vi "Line Settings FGV.vi"(8 "error in (no error)":errorcluster, 9 "Get/Set":enum16{"Set", "Get"}(ring), 10 "Line":T1={"Topic Name"="MyTopic", "Domain Id"=0, "Advanced Configuration"={"typeName"="", "key Name"=enum."<none>", "domainParticipantQoSProfile"="", "dataWriterQoSProfile"="", "forceArrayMapping?"=FALSE, "forceUnboundedString?"=FALSE, "forceExclusiveReader?"=FALSE, "forceRead? (only ExclusiveReader)"=FALSE, "ContentFilteredTopic Info"={"Filter Type"="DDS_SQLFILTER_NAME", "ContentFilteredTopic Name"="", "Filter Expression"=""}}}, 11 "Item Ref in":T5 format="%.0x") -> (0 "error out":errorcluster, 2 "Line":T1={"Topic Name"="MyTopic", "Domain Id"=0, "Advanced Configuration"={"typeName"="", "key Name"=enum."<none>", "domainParticipantQoSProfile"="", "dataWriterQoSProfile"="", "forceArrayMapping?"=FALSE, "forceUnboundedString?"=FALSE, "forceExclusiveReader?"=FALSE, "forceRead? (only ExclusiveReader)"=FALSE, "ContentFilteredTopic Info"={"Filter Type"="DDS_SQLFILTER_NAME", "ContentFilteredTopic Name"="", "Filter Expression"=""}}}, 3 "Item Ref out":T5=18446744073709551615 format="%.0x")   [LabVIEW 2016, in "DDS Custom Device System Explorer.lvlib"]
uses:
  DDS Custom Device System Explorer.lvlib
  <vilib>/NI Veristand/Custom Device API/Custom Device Item Ref.ctl
  Shared/WriterReaderConfiguration.ctl
  Shared/Advanced DDS Configuration.ctl
  Shared/key Enum.ctl
  <vilib>/RTI DDS Toolkit/Types/RTI DDS ContentFilteredTopic Info.ctl
  Shared/Constants.vi
  <vilib>/NI Veristand/Custom Device API/Set Item Property (U32).vi
  <vilib>/NI Veristand/Custom Device API/Set Item Property (String).vi
  <vilib>/NI Veristand/Custom Device API/Set Item Property (Boolean).vi
  <vilib>/NI Veristand/Custom Device API/Get Item Property (U32).vi
  <vilib>/NI Veristand/Custom Device API/Get Item Property (String).vi
  <vilib>/NI Veristand/Custom Device API/Get Item Property (Boolean).vi
  <vilib>/NI VeriStand/Custom Device API/Custom Device API.lvlib
  Shared/DDS Custom Device Shared.lvlib
  <vilib>/RTI DDS Toolkit/Library/LVDDS_library.lvlib
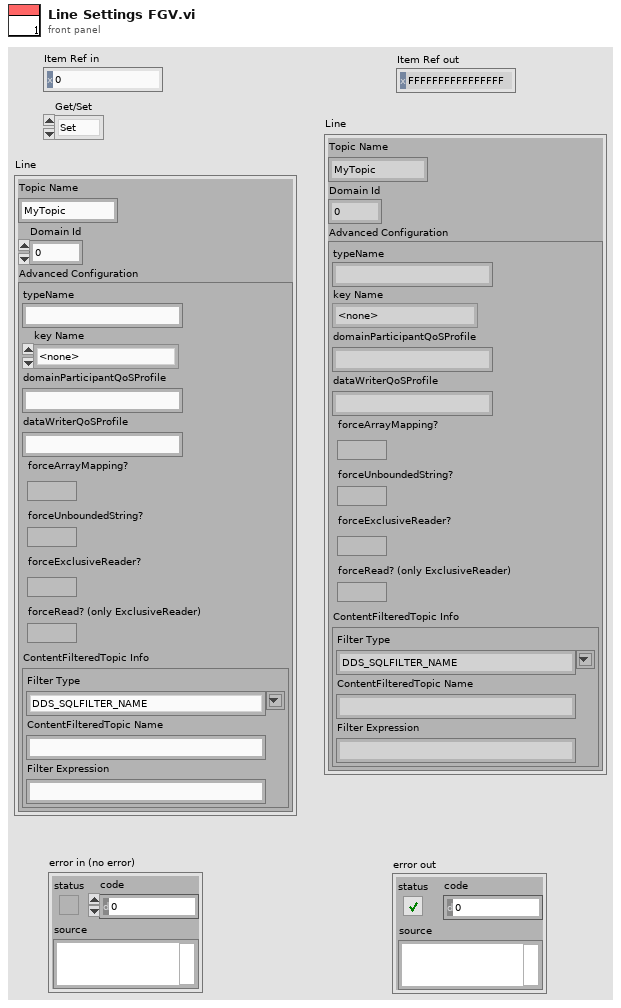
[diagram p1: front panel]
types:
  T1 = typedef "DDS Custom Device Shared.lvlib/WriterReaderConfiguration.ctl" = cluster{"Topic Name":string, "Domain Id":u32, "Advanced Configuration":T2}
  T2 = typedef "DDS Custom Device Shared.lvlib/Advanced DDS Configuration.ctl" = cluster{"typeName":string, "key Name":T3, "domainParticipantQoSProfile":string, "dataWriterQoSProfile":string, "forceArrayMapping?":bool, "forceUnboundedString?":bool, "forceExclusiveReader?":bool, "forceRead? (only ExclusiveReader)":bool, "ContentFilteredTopic Info":T4}
  T3 = typedef "DDS Custom Device Shared.lvlib/key Enum.ctl" = enum16{"<none>", "I32_Num", "I64_Num", "U16_Num", "innercluster.Sgl_Num", "innercluster.Boolean"}
  T4 = typedef "LVDDS_library.lvlib/RTI DDS ContentFilteredTopic Info.ctl" = cluster{"Filter Type":string, "ContentFilteredTopic Name":string, "Filter Expression":string}
  T5 = typedef "Custom Device API.lvlib/Custom Device Item Ref.ctl" = u64
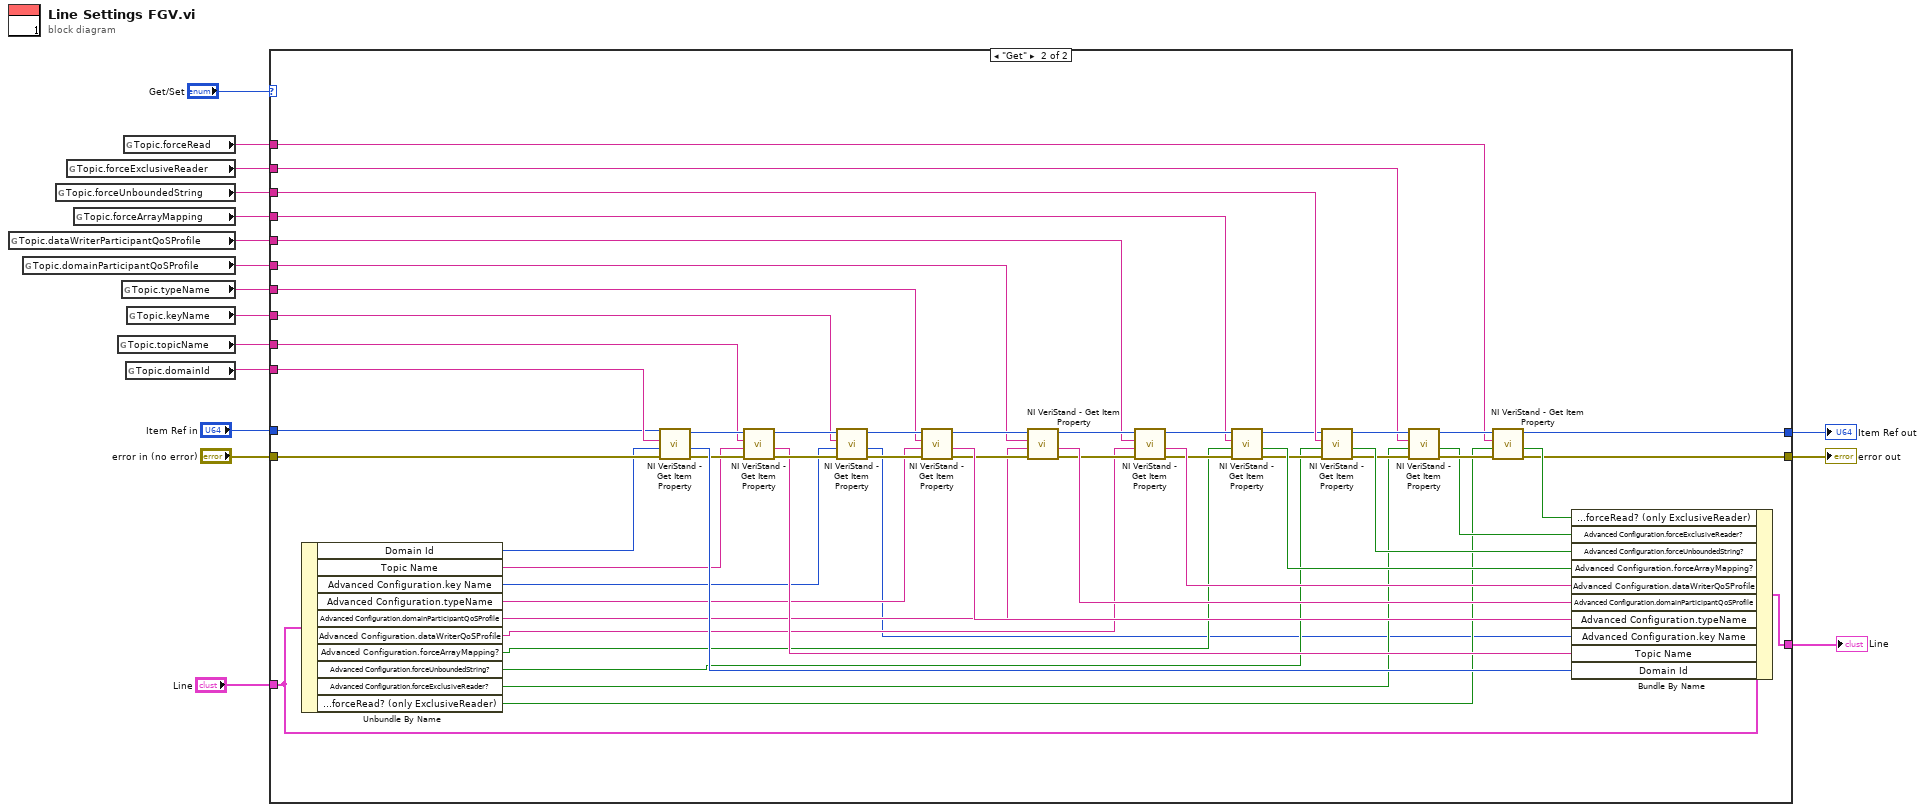
[diagram p0: block diagram]
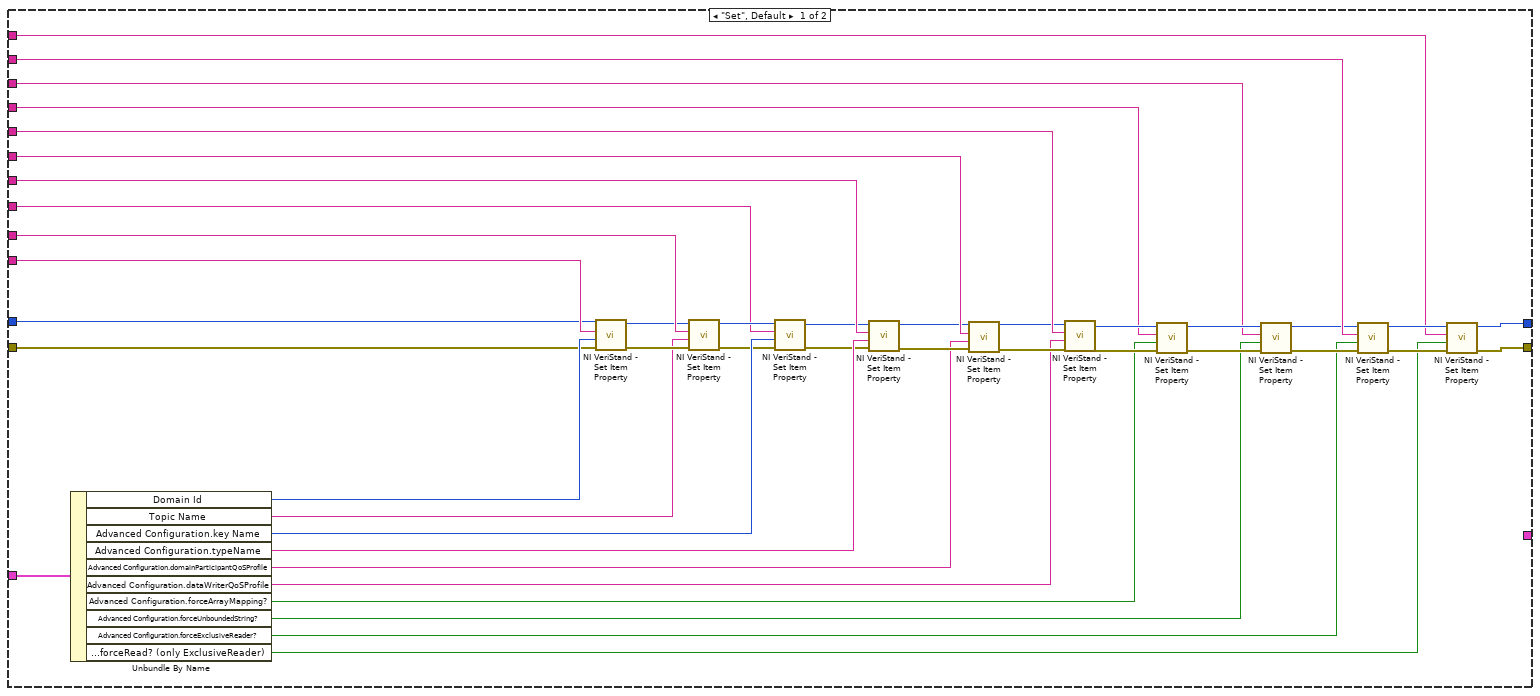
[diagram p2: hidden frame]
diagram:
  n1 = global read "Constants.vi" "Topic.dataWriterParticipantQoSProfile"() -> (w10:string)
  n2 = global read "Constants.vi" "Topic.domainParticipantQoSProfile"() -> (w11:string)
  n3 = global read "Constants.vi" "Topic.forceUnboundedString"() -> (w8:string)
  n4 = global read "Constants.vi" "Topic.forceExclusiveReader"() -> (w4:string)
  n5 = global read "Constants.vi" "Topic.forceArrayMapping"() -> (w9:string)
  n6 = global read "Constants.vi" "Topic.topicName"() -> (w14:string)
  n7 = global read "Constants.vi" "Topic.typeName"() -> (w13:string)
  n8 = global read "Constants.vi" "Topic.forceRead"() -> (w3:string)
  n9 = global read "Constants.vi" "Topic.domainId"() -> (w15:string)
  n10 = global read "Constants.vi" "Topic.keyName"() -> (w5:string)
  n11 = case shown="\"Get\"" "Get/Set" {
    tunnel: "error in (no error)" -> [w18 w73]
    tunnel: w15 -> [w60 w114]
    tunnel: w14 -> [w58 w110]
    tunnel: w13 -> [w57 w103]
    tunnel: "Item Ref in" -> [w19 w74]
    tunnel: w11 -> [w55 w99]
    tunnel: "Line" -> [w52 w72]
    tunnel: w10 -> [w47 w95]
    tunnel: w9 -> [w39 w91]
    tunnel: w8 -> [w38 w88]
    tunnel: [w25 w76] -> w6
    tunnel: [w26 w75] -> w7
    tunnel: w5 -> [w30 w106]
    tunnel: [_ w86] -> w1
    tunnel: w4 -> [w29 w80]
    tunnel: w3 -> [w21 w78]
    frame "Set", Default {
      n12 = Unbundle By Name(w52) -> ("Domain Id"=w51:u32, "Topic Name"=w50:string, "Advanced Configuration.key Name"=w35:T3, "Advanced Configuration.typeName"=w49:string, "Advanced Configuration.domainParticipantQoSProfile"=w48:string, "Advanced Configuration.dataWriterQoSProfile"=w44:string, "Advanced Configuration.forceArrayMapping?"=w37:bool, "Advanced Configuration.forceUnboundedString?"=w36:bool, "Advanced Configuration.forceExclusiveReader?"=w22:bool, "Advanced Configuration.forceRead? (only ExclusiveReader)"=w20:bool)
      n13 = call-poly <vilib>:"NI VeriStand - Set Item Property.vi"("error in (no error)"=w18, "Value"=w51, "Property Name"=w60, "Item Ref in"=w19) -> ("error out"=w59:errorcluster, "Item Ref out"=w56:T5)  [unwired: 5 in, 1 out]
      n14 = call-poly <vilib>:"NI VeriStand - Set Item Property.vi"("error in (no error)"=w59, "Value"=w50, "Property Name"=w58, "Item Ref in"=w56) -> ("error out"=w34:errorcluster, "Item Ref out"=w31:T5)  [unwired: 5 in, 1 out]
      n15 = call-poly <vilib>:"NI VeriStand - Set Item Property.vi"("error in (no error)"=w34, "Value"=w35, "Property Name"=w30, "Item Ref in"=w31) -> ("error out"=w33:errorcluster, "Item Ref out"=w32:T5)  [unwired: 5 in, 1 out]
      n16 = call-poly <vilib>:"NI VeriStand - Set Item Property.vi"("error in (no error)"=w33, "Value"=w49, "Property Name"=w57, "Item Ref in"=w32) -> ("error out"=w53:errorcluster, "Item Ref out"=w54:T5)  [unwired: 5 in, 1 out]
      n17 = call-poly <vilib>:"NI VeriStand - Set Item Property.vi"("error in (no error)"=w53, "Value"=w48, "Property Name"=w55, "Item Ref in"=w54) -> ("error out"=w45:errorcluster, "Item Ref out"=w46:T5)  [unwired: 5 in, 1 out]
      n18 = call-poly <vilib>:"NI VeriStand - Set Item Property.vi"("error in (no error)"=w45, "Value"=w44, "Property Name"=w47, "Item Ref in"=w46) -> ("error out"=w43:errorcluster, "Item Ref out"=w40:T5)  [unwired: 5 in, 1 out]
      n19 = call-poly <vilib>:"NI VeriStand - Set Item Property.vi"("error in (no error)"=w43, "Value"=w37, "Property Name"=w39, "Item Ref in"=w40) -> ("error out"=w42:errorcluster, "Item Ref out"=w41:T5)  [unwired: 5 in, 1 out]
      n20 = call-poly <vilib>:"NI VeriStand - Set Item Property.vi"("error in (no error)"=w42, "Value"=w36, "Property Name"=w38, "Item Ref in"=w41) -> ("error out"=w23:errorcluster, "Item Ref out"=w28:T5)  [unwired: 5 in, 1 out]
      n21 = call-poly <vilib>:"NI VeriStand - Set Item Property.vi"("error in (no error)"=w23, "Value"=w22, "Property Name"=w29, "Item Ref in"=w28) -> ("error out"=w24:errorcluster, "Item Ref out"=w27:T5)  [unwired: 5 in, 1 out]
      n22 = call-poly <vilib>:"NI VeriStand - Set Item Property.vi"("error in (no error)"=w24, "Value"=w20, "Property Name"=w21, "Item Ref in"=w27) -> ("error out"=w25:errorcluster, "Item Ref out"=w26:T5)  [unwired: 5 in, 1 out]
    }
    frame "Get" {
      n23 = Unbundle By Name(w72) -> ("Domain Id"=w71:u32, "Topic Name"=w70:string, "Advanced Configuration.key Name"=w69:T3, "Advanced Configuration.typeName"=w68:string, "Advanced Configuration.domainParticipantQoSProfile"=w67:string, "Advanced Configuration.dataWriterQoSProfile"=w66:string, "Advanced Configuration.forceArrayMapping?"=w65:bool, "Advanced Configuration.forceUnboundedString?"=w64:bool, "Advanced Configuration.forceExclusiveReader?"=w63:bool, "Advanced Configuration.forceRead? (only ExclusiveReader)"=w62:bool)
      n24 = call-poly <vilib>:"NI VeriStand - Get Item Property.vi"("error in (no error)"=w73, "Default Value"=w71, "Property Name"=w114, "Item Ref in"=w74) -> ("error out"=w112:errorcluster, "Value"=w113:u32, "Item Ref out"=w111:T5)  [unwired: 4 in, 1 out]
      n25 = call-poly <vilib>:"NI VeriStand - Get Item Property.vi"("error in (no error)"=w112, "Default Value"=w70, "Property Name"=w110, "Item Ref in"=w111) -> ("error out"=w109:errorcluster, "Value"=w107:string, "Item Ref out"=w108:T5)  [unwired: 4 in, 1 out]
      n26 = call-poly <vilib>:"NI VeriStand - Get Item Property.vi"("error in (no error)"=w109, "Default Value"=w69, "Property Name"=w106, "Item Ref in"=w108) -> ("error out"=w105:errorcluster, "Value"=w61:u32, "Item Ref out"=w104:T5)  [unwired: 4 in, 1 out]
      n27 = call-poly <vilib>:"NI VeriStand - Get Item Property.vi"("error in (no error)"=w105, "Default Value"=w68, "Property Name"=w103, "Item Ref in"=w104) -> ("error out"=w101:errorcluster, "Value"=w102:string, "Item Ref out"=w100:T5)  [unwired: 4 in, 1 out]
      n28 = call-poly <vilib>:"NI VeriStand - Get Item Property.vi"("error in (no error)"=w101, "Default Value"=w67, "Property Name"=w99, "Item Ref in"=w100) -> ("error out"=w96:errorcluster, "Value"=w98:string, "Item Ref out"=w97:T5)  [unwired: 4 in, 1 out]
      n29 = call-poly <vilib>:"NI VeriStand - Get Item Property.vi"("error in (no error)"=w96, "Default Value"=w66, "Property Name"=w95, "Item Ref in"=w97) -> ("error out"=w93:errorcluster, "Value"=w94:string, "Item Ref out"=w92:T5)  [unwired: 4 in, 1 out]
      n30 = call-poly <vilib>:"NI VeriStand - Get Item Property.vi"("error in (no error)"=w93, "Default Value"=w65, "Property Name"=w91, "Item Ref in"=w92) -> ("error out"=w89:errorcluster, "Value"=w90:bool, "Item Ref out"=w87:T5)  [unwired: 4 in, 1 out]
      n31 = call-poly <vilib>:"NI VeriStand - Get Item Property.vi"("error in (no error)"=w89, "Default Value"=w64, "Property Name"=w88, "Item Ref in"=w87) -> ("error out"=w84:errorcluster, "Value"=w85:bool, "Item Ref out"=w81:T5)  [unwired: 4 in, 1 out]
      n32 = call-poly <vilib>:"NI VeriStand - Get Item Property.vi"("error in (no error)"=w84, "Default Value"=w63, "Property Name"=w80, "Item Ref in"=w81) -> ("error out"=w83:errorcluster, "Value"=w79:bool, "Item Ref out"=w82:T5)  [unwired: 4 in, 1 out]
      n33 = call-poly <vilib>:"NI VeriStand - Get Item Property.vi"("error in (no error)"=w83, "Default Value"=w62, "Property Name"=w78, "Item Ref in"=w82) -> ("error out"=w76:errorcluster, "Value"=w77:bool, "Item Ref out"=w75:T5)  [unwired: 4 in, 1 out]
      n34 = Bundle By Name(cluster=w72, "Advanced Configuration.forceRead? (only ExclusiveReader)"=w77, "Advanced Configuration.forceExclusiveReader?"=w79, "Advanced Configuration.forceUnboundedString?"=w85, "Advanced Configuration.forceArrayMapping?"=w90, "Advanced Configuration.dataWriterQoSProfile"=w94, "Advanced Configuration.domainParticipantQoSProfile"=w98, "Advanced Configuration.typeName"=w102, "Advanced Configuration.key Name"=w61, "Topic Name"=w107, "Domain Id"=w113) -> (w86:T1)
    }
  }
  "Item Ref out" <- w7
  "error out" <- w6
  "Line" <- w1
